vi "TveFeRfe.vi"(8 "error in (no error)":errorcluster, 11 "PmuAnalysis in":refnum<class "PmuAnalysis.lvclass">) -> (0 "error out":errorcluster, 3 "PmuAnalysis out":refnum<class "PmuAnalysis.lvclass">)   [LabVIEW 2014, in "AnalysisPlugins.lvlib" / "PmuAnalysis.lvclass"]
uses:
  PmuAnalysis.lvclass
  <vilib>/Analysis/NI_AAL_Angle.lvlib
  <vilib>/Analysis/coordinate.llb/Wrap Angle (scalar).vi
  <vilib>/Analysis/coordinate.llb/Angle Range (Degree).ctl
  <vilib>/Analysis/coordinate.llb/Angle Units.ctl
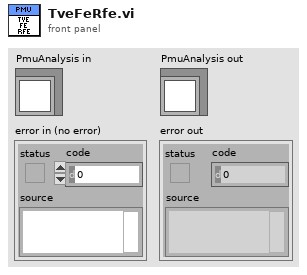
[diagram p1: front panel]
types:
  T1 = typedef "AnalysisPlugins.lvlib/PmuAnalysis.lvclass/PmuData.ctl" = cluster{"Timestamp":dbl, "Synx":cdb[], "Freq":dbl, "ROCOF":dbl, "ID":i16}
  T2 = typedef "NI_AAL_Angle.lvlib/Angle Units.ctl" = i32
  T3 = typedef "NI_AAL_Angle.lvlib/Angle Range (Degree).ctl" = u16
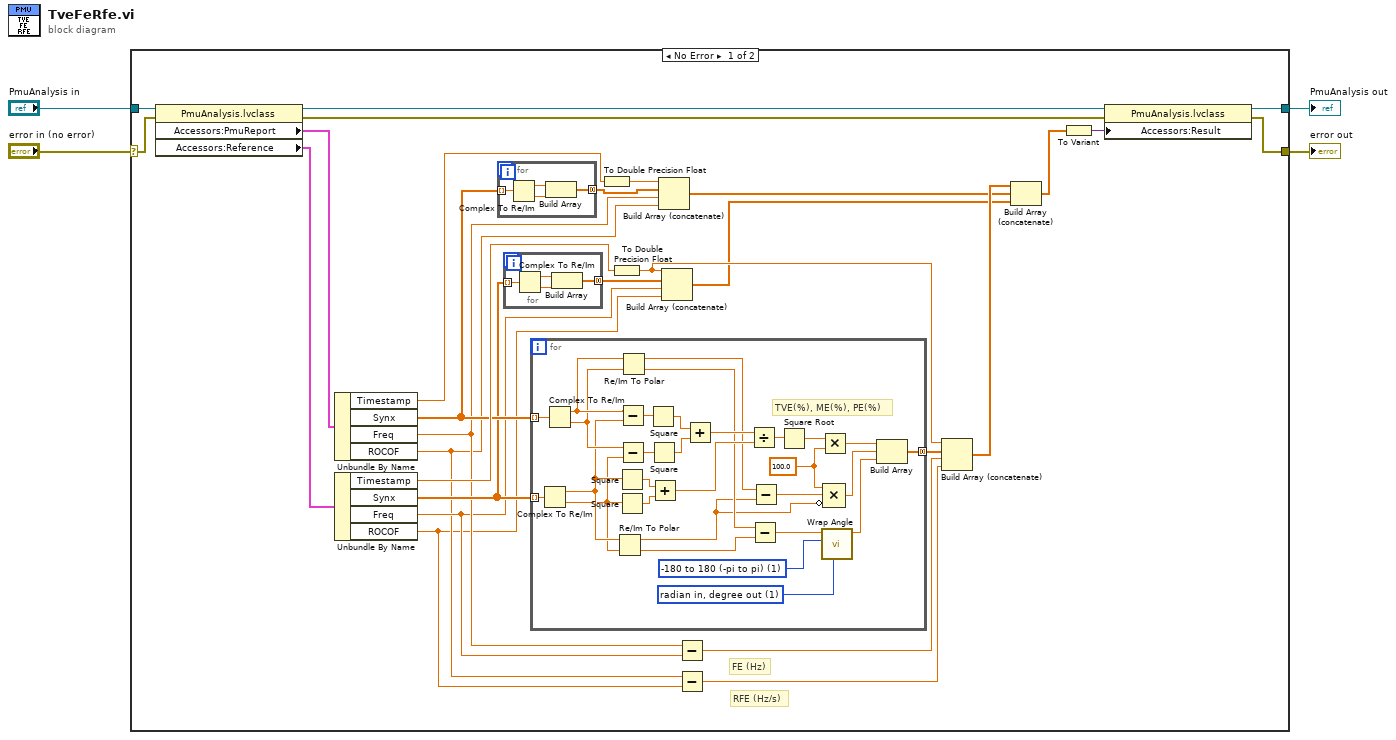
[diagram p0: block diagram]
diagram:
  n1 = case shown="No Error" "error in (no error)" {
    selector: "error in (no error)" -> [w9 w71]
    tunnel: [w7 w71] -> w3
    tunnel: [w10 w70] -> w1
    tunnel: "PmuAnalysis in" -> [w32 w70]
    frame No Error {
      # "RFE (Hz/s)"
      # "FE (Hz)"
      n2 = property class="PmuAnalysis.lvclass"(reference=w32, error in=w9) -> (reference out=w31:refnum<class "PmuAnalysis.lvclass">, error out=w8:errorcluster, "Accessors:PmuReport"=w29:T1, "Accessors:Reference"=w30:T1)
      n3 = Unbundle By Name(w29) -> ("Timestamp"=w26:dbl, "Synx"=w23:cdb[], "Freq"=w19:dbl, "ROCOF"=w17:dbl)
      n4 = Unbundle By Name(w30) -> ("Timestamp"=w24:dbl, "Synx"=w22:cdb[], "Freq"=w18:dbl, "ROCOF"=w16:dbl)
      n5 = for {
        tunnel: w23 -> [w69] mode=indexing
        tunnel: [w66] -> w27 mode=concatenating
        n6 = Complex To Re/Im(x + iy=w69) -> (x=w68:dbl, y=w67:dbl)
        n7 = Build Array(w68, w67) -> (w66:dbl[])
      }
      n8 = for {
        tunnel: [w63] -> w25 mode=concatenating
        tunnel: w22 -> [w62] mode=indexing
        n9 = Complex To Re/Im(x + iy=w62) -> (x=w65:dbl, y=w64:dbl)
        n10 = Build Array(w65, w64) -> (w63:dbl[])
      }
      n11 = for {
        tunnel: w23 -> [w61] mode=indexing
        tunnel: w22 -> [w60] mode=indexing
        tunnel: [w33] -> w20 mode=concatenating
        w37 = T2 1 items=["radian in, radian out", "radian in, degree out", "degree in, degree out", "degree in, radian out"] ("angle units")
        w38 = T3 1 items=["none", "-180 to 180 (-pi to pi)", "0 to 360 (0 to 2pi)"] ("angle range")
        w40 = 100.0 ("y")
        # "TVE(%), ME(%), PE(%)"
        n12 = Complex To Re/Im(x + iy=w60) -> (x=w49:dbl, y=w48:dbl)
        n13 = Complex To Re/Im(x + iy=w61) -> (x=w59:dbl, y=w58:dbl)
        n14 = Re/Im To Polar(2:w48, 3:w49) -> (0:w44:dbl, 1:w42:dbl)
        n15 = Square(x=w49) -> (x^2=w51:dbl)
        n16 = Square(x=w48) -> (x^2=w52:dbl)
        n17 = Subtract(x=w59, y=w49) -> (x-y=w57:dbl)
        n18 = Subtract(x=w58, y=w48) -> (x-y=w56:dbl)
        n19 = Re/Im To Polar(2:w58, 3:w59) -> (0:w45:dbl, 1:w46:dbl)
        n20 = Square(x=w57) -> (x^2=w55:dbl)
        n21 = Square(x=w56) -> (x^2=w54:dbl)
        n22 = Add(x=w51, y=w52) -> (x+y=w50:dbl)
        n23 = Add(x=w55, y=w54) -> (x+y=w53:dbl)
        n24 = Divide(x=w53, y=w50) -> (x/y=w47:dbl)
        n25 = Subtract(x=w45, y=w44) -> (x-y=w39:dbl)
        n26 = Subtract(x=w46, y=w42) -> (x-y=w43:dbl)
        n27 = Square Root(x=w47) -> (sqrt(x)=w41:dbl)
        n28 = Multiply(x=w41, y=w40) -> (x*y=w36:dbl)
        n29 = call-poly <vilib>:"Wrap Angle.vi"("angle units"=w37, "angle range"=w38, "angle in"=w39) -> ("angle out"=w34:dbl)  [unwired: 7 in, 1 out]
        n30 = Compound Arithmetic op=MULTIPLY(w40, w43, invert w42) -> (w35:dbl)
        n31 = Build Array(w36, w35, w34) -> (w33:dbl[])
      }
      n32 = To Double Precision Float(number=w26) -> (double precision float=w28:dbl)
      n33 = To Double Precision Float(number=w24) -> (double precision float=w21:dbl)
      n34 = Build Array (concatenate)(w28, w27, w19, w17) -> (w12:dbl[])
      n35 = Build Array (concatenate)(w21, w25, w18, w16) -> (w11:dbl[])
      n36 = Subtract(x=w19, y=w18) -> (x-y=w15:dbl)
      n37 = Subtract(x=w17, y=w16) -> (x-y=w14:dbl)
      n38 = Build Array (concatenate)(w21, w20, w15, w14) -> (w13:dbl[])
      n39 = Build Array (concatenate)(w13, w12, w11) -> (w6:dbl[])
      n40 = To Variant(anything=w6) -> (Variant=w5:variant)
      n41 = property class="PmuAnalysis.lvclass"(reference=w31, error in=w8, "Accessors:Result"=w5) -> (reference out=w10:refnum<class "PmuAnalysis.lvclass">, error out=w7:errorcluster)
    }
    frame Error {
    }
  }
  "error out" <- w3
  "PmuAnalysis out" <- w1
